vi "ClearServers.vi"(1 "Clear Servers?":bool) -> (0 "Deleted Files":string[](array[string]))   [LabVIEW 2012]
doc: "Deletes topic servers from the servers folder so that they are respawned from _BlankServer.vi. Useful when changing _BlankServer implementation. \n\nWARNING: Do not inadvertently move this file. May delete all vi's if run from a different location."
panel:
  # "DO NOT MOVE THIS VI AROUND WITHOUT CHANGING THE FILE PATH!\nWILL DELETE ALL *.VI FILES THAT ARE NOT NAMED _BlankServer.vi"
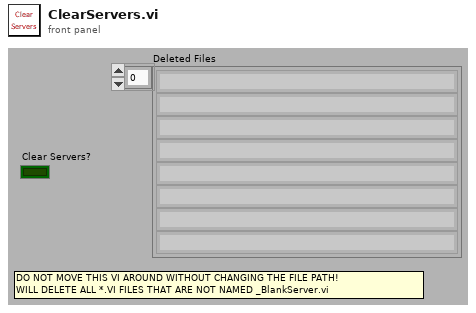
[diagram p1: front panel]
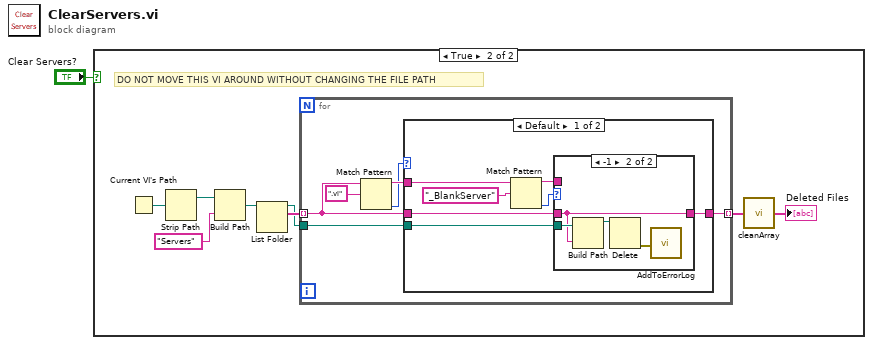
[diagram p0: block diagram]
diagram:
  n1 = case shown="True" "Clear Servers?" {
    frame False {
    }
    frame True {
      # "DO NOT MOVE THIS VI AROUND WITHOUT CHANGING THE FILE PATH"
      n2 = Current VI's Path() -> (path=w9:path)
      n3 = Strip Path(path=w9) -> (stripped path=w8:path)  [unwired: 1 out]
      n4 = Build Path(base path=w8, name or relative path="Servers") -> (appended path=w6:path)
      n5 = List Folder(path=w6) -> (path out=w4:path, filenames=w5:string[])  [unwired: 3 in, 2 out]
      n6 = for {
        tunnel: w5 -> [w12] mode=indexing
        tunnel: w4 -> [w13]
        tunnel: [w11] -> w3 mode=indexing
        n7 = Match Pattern(string=w12, regular expression=".vi") -> (before substring=w14:string, offset past match=w10:i32)  [unwired: 1 in, 2 out]
        n8 = case shown="Default" w10 {
          tunnel: w14 -> [w22 _]
          tunnel: w13 -> [w19 _]
          tunnel: w12 -> [w17 _]
          tunnel: [w16 _] -> w11
          frame Default {
            n9 = Match Pattern(string=w22, regular expression="_BlankServer") -> (before substring=w18:string, offset past match=w20:i32)  [unwired: 1 in, 2 out]
            n10 = case shown="-1" w20 {
              tunnel: w19 -> [_ w26]
              tunnel: w18 -> [_ _]
              tunnel: w17 -> [_ w25]
              tunnel: [_ w25] -> w16
              frame Default {
              }
              frame -1 {
                n11 = Build Path(base path=w26, name or relative path=w25) -> (appended path=w24:path)
                n12 = Delete(path (use dialog)=w24) -> (error out=w23:errorcluster)  [unwired: 4 in, 2 out]
                n13 = call <userlib>:"AddToErrorLog.vi"("error out"=w23) -> ()  [unwired: 1 in]
              }
            }
          }
          frame -1 {
            # "Don't delete non-labview files"
          }
        }
      }
      n14 = call <userlib>:"cleanArray.vi"("Array in"=w3) -> ("Array out"=→"Deleted Files":string[])
    }
  }
